vi "micImport.vi"(11 "mic data":path) -> (1 "mic data":cluster{dbl[][], dbl[][]}, 2 "I_660, mV":dbl[][](array[numeric]), 3 "I_532, mV":dbl[][](array[numeric]))   [LabVIEW 2011]
uses:
  <vilib>/Utility/file.llb/Read From Spreadsheet File (DBL).vi
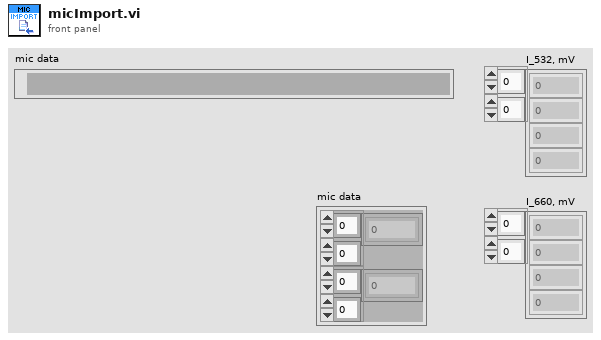
[diagram p1: front panel]
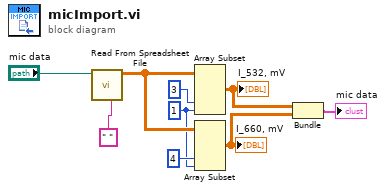
[diagram p0: block diagram]
diagram:
  w7 = 1 ("length")
  n1 = call-poly <vilib>:"Read From Spreadsheet File.vi"("delimiter (\\t)"=" " ("delimiter (\\t)"), "file path (dialog if empty)"="mic data") -> ("all rows"=w9:dbl[][])  [unwired: 5 in, 4 out]
  n2 = Array Subset(array=w9, index (col)=3 ("index"), length (col)=w7) -> (w3:dbl[][])  [unwired: 2 in]
  "I_532, mV" <- w3
  n3 = Array Subset(array=w9, index (col)=4 ("index"), length (col)=w7) -> (w2:dbl[][])  [unwired: 2 in]
  "I_660, mV" <- w2
  n4 = Bundle(w3, w2) -> (→"mic data":cluster{dbl[][], dbl[][]})  [unwired: 1 in]
